vi "Ch_setup_string.vi"(6 "Analysis Info cluster":T1[](array[typedef]) {"Sync Delay Time (s)" format="%.4f"; "Sd Error in Variance" format="%.2f"; "Skew_u" format="%.2f"; "% u'/U" format="%.2f"; "Sd Error in Mean" format="%.2f"; "Kurt_u" format="%.2f"; "u^4" format="%.2f"; "u^3" format="%.2f"; "U" format="%.2f"; "u^2" format="%.2f"}) -> (1 "Output string":string)   [LabVIEW 2020]
uses:
  Controls/Analysis_info_cluster.ctl
  Controls/Inst_type.ctl
  Controls/Instrument_Array.ctl
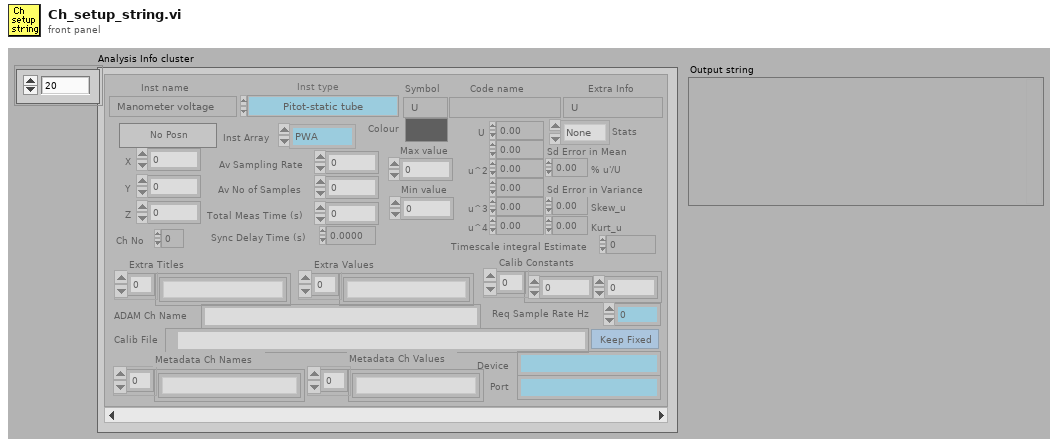
[diagram p1: front panel]
types:
  T1 = typedef "Analysis_info_cluster.ctl" = cluster{"Colour":u32, "Inst type":T2, "Inst name":string, "Symbol":string, "Code name":string, "Extra Info":string, "Inst Array":T3, "Extra Titles":string[], "Extra Values":string[], "U":dbl, "u^2":dbl, "u^3":dbl, "u^4":dbl, "Skew_u":dbl, "Kurt_u":dbl, "Sd Error in Mean":dbl, "% u'/U":dbl, "X":dbl, "Y":dbl, "Z":dbl, "Timescale integral Estimate":dbl, "Sd Error in Variance":dbl, "Calib File":path, "Calib Constants":dbl[], "Output Position":bool, "Stats":enum16{"None", "Basic", "Full"}, "Av Sampling Rate":dbl, "Av No of Samples":dbl, "Total Meas Time (s)":dbl, "ADAM Ch Name":string, "Max value":dbl, "Min value":dbl, "Req Sample Rate Hz":dbl, "Sync Delay Time (s)":dbl, "Ch No":i16, "Device":string, "Use Latest Calib":bool, "Port":string, "Metadata Ch Names":string[], "Metadata Ch Values":string[]}
  T2 = typedef "Inst_type.ctl" = enum16{"Propeller anemometer", "Raw voltage", "Pressure Transducer", "Pitot-static tube", "Preston tube", "Hot wire", "Cross wire 1", "Cross wire 2", "Generic Linear", "Generic Polynomial", "Generic BackPoly", "Fast FID", "Thermocouple", "Cold wire", "Pulsed Wire", "LDA Vel", "LDA Tran time", "LDA Arr time", "Microphone"}
  T3 = typedef "Instrument_Array.ctl" = enum16{"PWA", "LDA", "Analogue"}
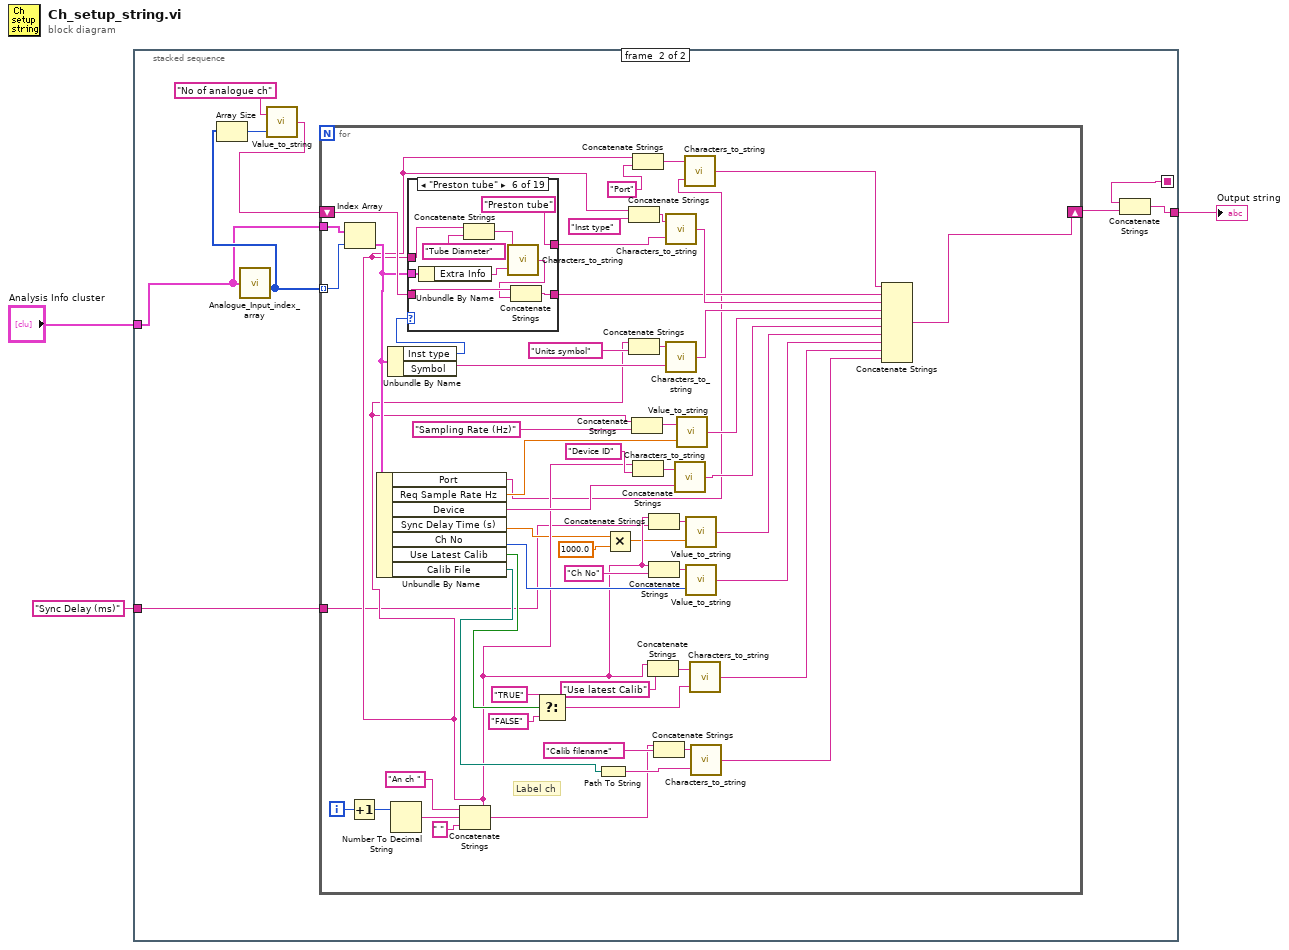
[diagram p0: block diagram]
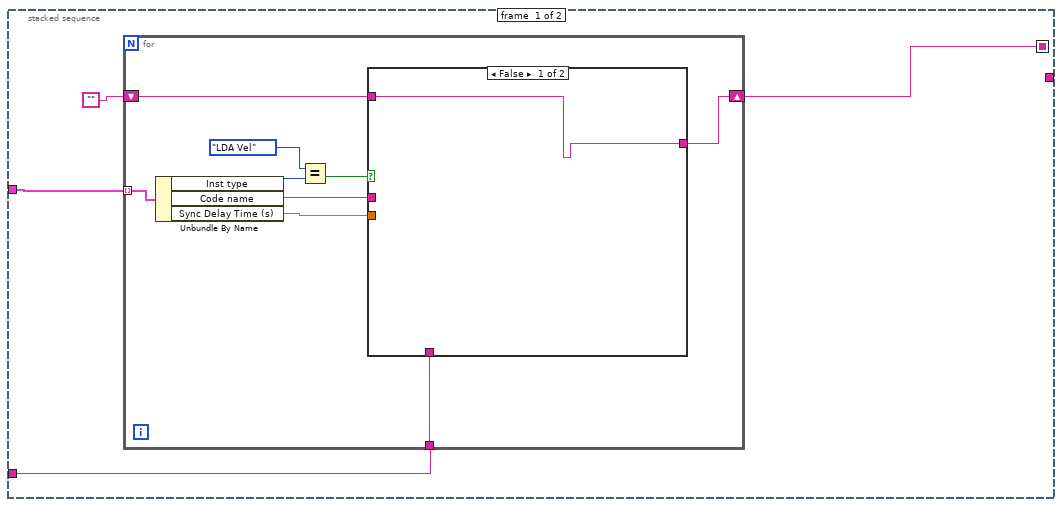
[diagram p2: hidden frame]
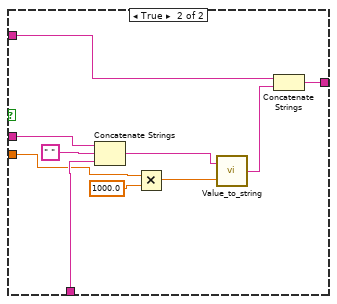
[diagram p3: hidden frame]
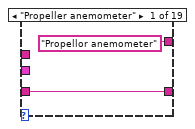
[diagram p4: hidden frame]
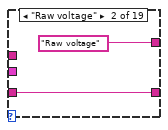
[diagram p5: hidden frame]
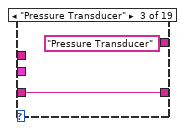
[diagram p6: hidden frame]
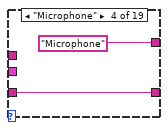
[diagram p7: hidden frame]
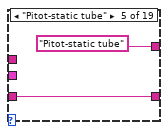
[diagram p8: hidden frame]
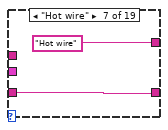
[diagram p9: hidden frame]
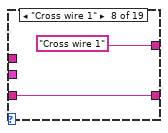
[diagram p10: hidden frame]
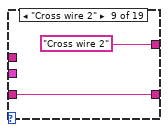
[diagram p11: hidden frame]
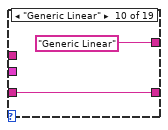
[diagram p12: hidden frame]
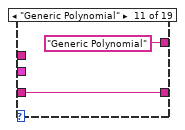
[diagram p13: hidden frame]
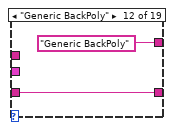
[diagram p14: hidden frame]
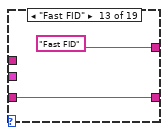
[diagram p15: hidden frame]
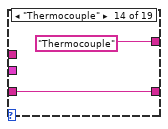
[diagram p16: hidden frame]
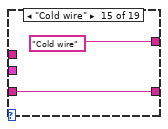
[diagram p17: hidden frame]
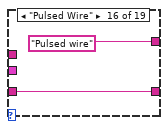
[diagram p18: hidden frame]
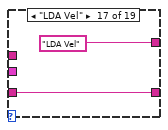
[diagram p19: hidden frame]
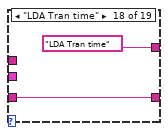
[diagram p20: hidden frame]
diagram:
  n1 = stacked-sequence {
    seq-local: [w4 _] -> [_ w29]
    tunnel: [_ w28] -> w3
    tunnel: "Analysis Info cluster" -> [w7 w32]
    tunnel: "Sync Delay (ms)" -> [w6 w31]
    frame #0 {
      n2 = for {
        tunnel: w7 -> [w16] mode=indexing
        tunnel: w6 -> [w12]
        shift-right: [w9] -> w4
        shift-left: "" -> [w10]
        n3 = Unbundle By Name(w16) -> ("Inst type"=w15:T2, "Code name"=w13:string, "Sync Delay Time (s)"=w11:dbl)
        n4 = Equal?(x=Inst_type."LDA Vel" ("Inst type"), y=w15) -> (x = y?=w8:bool)
        n5 = case shown="False" w8 {
          tunnel: w13 -> [_ w25]
          tunnel: w12 -> [_ w24]
          tunnel: w11 -> [_ w21]
          tunnel: w10 -> [w17 w19]
          tunnel: [w17 w18] -> w9
          frame False {
          }
          frame True {
            n6 = Concatenate Strings(w25, " " ("string"), w24) -> (w22:string)
            n7 = Multiply(x=w21, y=1000.0) -> (x*y=w27:dbl)
            n8 = call "Value_to_string.vi"("Value"=w27, "Label for value"=w22) -> ("Output string"=w20:string)  [unwired: 1 in]
            n9 = Concatenate Strings(w19, w20) -> (w18:string)
          }
        }
      }
    }
    frame #1 {
      n10 = call "Analogue_Input_index_array.vi"("Analysis Info cluster"=w32) -> ("Array"=w35:i32[])
      n11 = Array Size(array=w35) -> (size(s)=w34:i32)
      n12 = call "Value_to_string.vi"("Value"=w34, "Label for value"="No of analogue ch") -> ("Output string"=w33:string)  [unwired: 1 in]
      n13 = for {
        shift-right: [w91] -> w30
        shift-left: w33 -> [w82]
        tunnel: w32 -> [w79]
        tunnel: w35 -> [w78] mode=indexing
        tunnel: w31 -> [w37]
        i -> [w51]
        # "Label ch"
        n14 = Index Array(array=w79, index=w78) -> (element=w61:T1)
        n15 = Increment(x=w51) -> (x+1=w55:i32)
        n16 = Unbundle By Name(w61) -> ("Port"=w43:string, "Req Sample Rate Hz"=w77:dbl, "Device"=w75:string, "Sync Delay Time (s)"=w40:dbl, "Ch No"=w69:i16, "Use Latest Calib"=w72:bool, "Calib File"=w47:path)
        n17 = Unbundle By Name(w61) -> ("Inst type"=w80:T2, "Symbol"=w90:string)
        n18 = Number To Decimal String(number=w55) -> (decimal integer string=w54:string)  [unwired: 1 out]
        n19 = Concatenate Strings("An ch ", w54, " ") -> (w45:string)
        n20 = case shown="\"Preston tube\"" w80 {
          tunnel: ["Propellor anemometer" "Raw voltage" "Pressure Transducer" "Microphone" "Pitot-static tube" "Preston tube" "Hot wire" "Cross wire 1" "Cross wire 2" "Generic Linear" "Generic Polynomial" "Generic BackPoly" "Fast FID" "Thermocouple" "Cold wire" "Pulsed wire" "LDA Vel" "LDA Tran time" "LDA Arr time"] -> w89
          tunnel: w82 -> [w92 w94 w96 w98 w100 w108 w111 w113 w115 w117 w119 w121 w123 w125 w127 w129 w131 w133 w135]
          tunnel: [w92 w94 w96 w98 w100 w107 w111 w113 w115 w117 w119 w121 w123 w125 w127 w129 w131 w133 w135] -> w81
          tunnel: w61 -> [_ _ _ _ _ w110 _ _ _ _ _ _ _ _ _ _ _ _ _]
          tunnel: w45 -> [_ _ _ _ _ w103 _ _ _ _ _ _ _ _ _ _ _ _ _]
          frame "Propeller anemometer" {
          }
          frame "Raw voltage" {
          }
          frame "Pressure Transducer" {
          }
          frame "Microphone" {
          }
          frame "Pitot-static tube" {
          }
          frame "Preston tube" {
            n21 = Unbundle By Name(w110) -> ("Extra Info"=w109:string)
            n22 = Concatenate Strings(w103, "Tube Diameter") -> (w102:string)
            n23 = call "Characters_to_string.vi"("Characters to write"=w109, "Label for characters"=w102) -> ("Output string"=w105:string)  [unwired: 1 in]
            n24 = Concatenate Strings(w108, w105) -> (w107:string)
          }
          frame "Hot wire" {
          }
          frame "Cross wire 1" {
          }
          frame "Cross wire 2" {
          }
          frame "Generic Linear" {
          }
          frame "Generic Polynomial" {
          }
          frame "Generic BackPoly" {
          }
          frame "Fast FID" {
          }
          frame "Thermocouple" {
          }
          frame "Cold wire" {
          }
          frame "Pulsed Wire" {
          }
          frame "LDA Vel" {
          }
          frame "LDA Tran time" {
          }
          frame "LDA Arr time" {
          }
        }
        n25 = Select(t="TRUE", s=w72, f="FALSE") -> (s? t:f=w71:string)
        n26 = Path To String(path=w47) -> (string=w50:string)
        n27 = Multiply(x=w40, y=1000.0) -> (x*y=w39:dbl)
        n28 = Concatenate Strings(w45, "Inst type") -> (w83:string)
        n29 = Concatenate Strings(w45, "Units symbol") -> (w84:string)
        n30 = Concatenate Strings(w45, "Sampling Rate (Hz)") -> (w76:string)
        n31 = Concatenate Strings(w45, "Port") -> (w44:string)
        n32 = Concatenate Strings(w45, "Device ID") -> (w73:string)
        n33 = Concatenate Strings(w45, "Use latest Calib") -> (w70:string)
        n34 = Concatenate Strings(w45, w37) -> (w74:string)
        n35 = Concatenate Strings(w45, "Ch No") -> (w68:string)
        n36 = Concatenate Strings(w45, "Calib filename") -> (w49:string)
        n37 = call "Characters_to_string.vi"("Characters to write"=w89, "Label for characters"=w83) -> ("Output string"=w85:string)  [unwired: 1 in]
        n38 = call "Characters_to_string.vi"("Characters to write"=w90, "Label for characters"=w84) -> ("Output string"=w86:string)  [unwired: 1 in]
        n39 = call "Characters_to_string.vi"("Characters to write"=w75, "Label for characters"=w73) -> ("Output string"=w59:string)  [unwired: 1 in]
        n40 = call "Value_to_string.vi"("Value"=w77, "Label for value"=w76) -> ("Output string"=w60:string)  [unwired: 1 in]
        n41 = call "Characters_to_string.vi"("Characters to write"=w43, "Label for characters"=w44) -> ("Output string"=w42:string)  [unwired: 1 in]
        n42 = call "Value_to_string.vi"("Value"=w39, "Label for value"=w74) -> ("Output string"=w58:string)  [unwired: 1 in]
        n43 = call "Value_to_string.vi"("Value"=w69, "Label for value"=w68) -> ("Output string"=w57:string)  [unwired: 1 in]
        n44 = call "Characters_to_string.vi"("Characters to write"=w71, "Label for characters"=w70) -> ("Output string"=w56:string)  [unwired: 1 in]
        n45 = call "Characters_to_string.vi"("Characters to write"=w50, "Label for characters"=w49) -> ("Output string"=w46:string)  [unwired: 1 in]
        n46 = Concatenate Strings(w42, w81, w85, w86, w60, w59, w58, w57, w56, w46) -> (w91:string)
      }
      n47 = Concatenate Strings(w29, w30) -> (w28:string)
    }
  }
  "Output string" <- w3
